vi "1D Weighted-Unweighted Chi2.vi"(8 "error in (no error)":errorcluster, 9 "Weight Array":dbl[](array[numeric]), 10 "Y Array":dbl[](array[numeric]), 11 "Fit Output":T1) -> (0 "error out":errorcluster, 3 "NL Fit Output":T1)   [LabVIEW 2021, in "Fits.lvlib"]
uses:
  Fits.lvlib
  Non-linear Fit Output v4.ctl
  Nonlinear Fit Method.ctl
  <vilib>/Analysis/Matrix/Datatypes/RealMatrix.ctl
  Convergence Criteria.ctl
  Non-linear Fitting Algorithm.ctl
  IRF(X)PSED/Fit Weights Type v2.ctl
  Graphs/XY Graph/XY Graph Plot Data.ctl
  <vilib>/Utility/error.llb/Error Cluster From Error Code.vi
  <vilib>/ErrorRing/Error Ring.xnode
  <vilib>/Analysis/Matrix/NI_Matrix.lvlib
  Graphs/XY Graph/XY Graph Add-Ons.lvlib
panel:
  # "see the AlliGator License on the block diagram (Ctrl+E or Window:Show Block Diagram)"
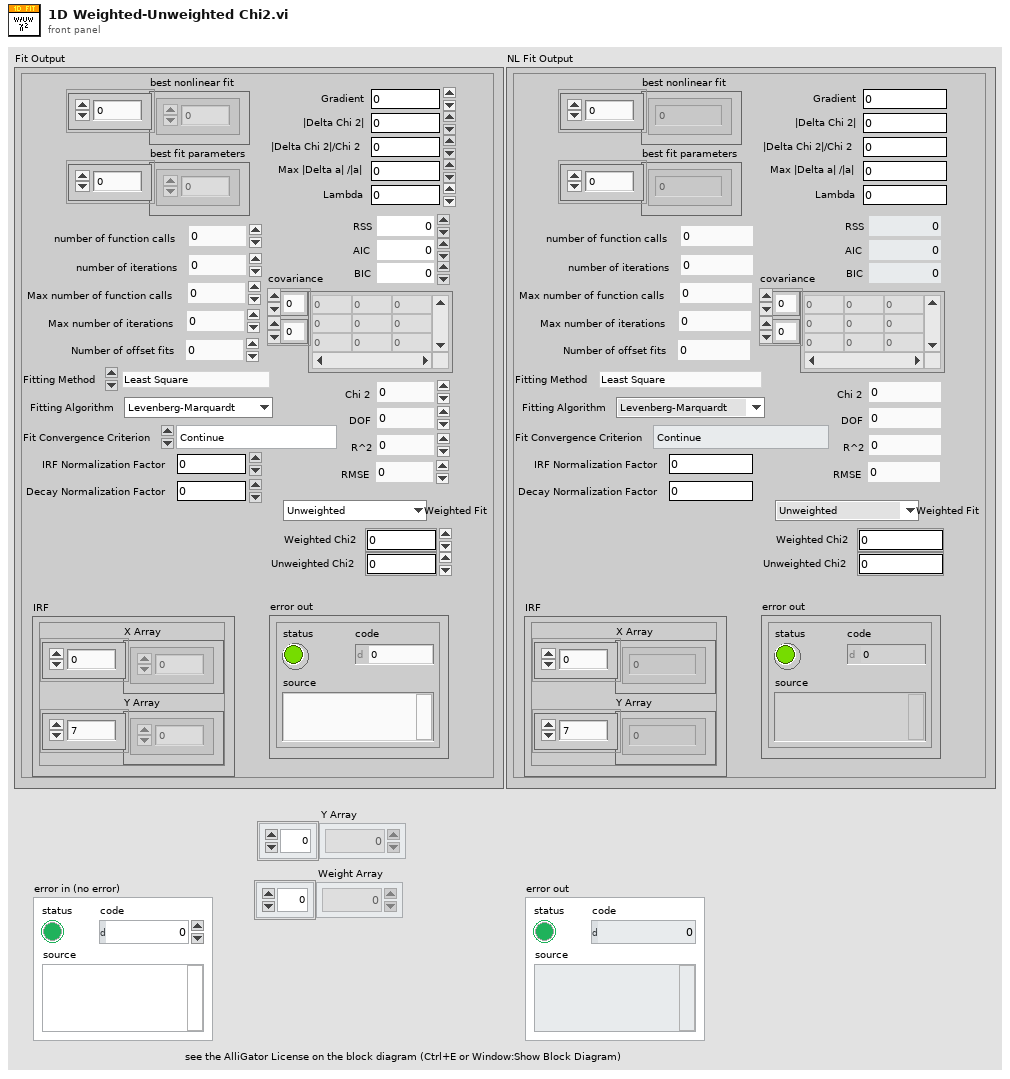
[diagram p1: front panel]
types:
  T1 = typedef "Fits.lvlib/Non-linear Fit Output v4.ctl" = cluster{"best nonlinear fit":dbl[], "best fit parameters":dbl[], "R^2":dbl, "RMSE":dbl, "error out":errorcluster, "Fitting Method":T2, "number of function calls":i32, "number of iterations":i32, "covariance":T3, "Chi 2":dbl, "DOF":i32, "Fit Convergence Criterion":T4, "Fitting Algorithm":T5, "Weighted Fit":T6, "Gradient":dbl, "|Delta Chi 2|":dbl, "|Delta Chi 2|/Chi 2":dbl, "Max |Delta a| /|a|":dbl, "Lambda":dbl, "RSS":dbl, "AIC":dbl, "BIC":dbl, "Max number of function calls":i32, "Max number of iterations":i32, "IRF":T7, "IRF Normalization Factor":dbl, "Decay Normalization Factor":dbl, "Number of offset fits":i32, "Weighted Chi2":dbl, "Unweighted Chi2":dbl}
  T2 = typedef "Fits.lvlib/Nonlinear Fit Method.ctl" = enum16{"Least Square", "Least Absolute Residual", "Bisquare", "MLE"}
  T3 = typedef "NI_Matrix.lvlib/RealMatrix.ctl" = dbl[][]
  T4 = typedef "Fits.lvlib/Convergence Criteria.ctl" = enum16{"Continue", "Tolerances Exceeded", "Max Time Exceeded", "Max Iterations Exceeded", "Max Function Evaluations Exceeded", "Scale Range Exceeded"}
  T5 = typedef "Fits.lvlib/Non-linear Fitting Algorithm.ctl" = enum16{"Levenberg-Marquardt", "Trust-Region Dogleg"}
  T6 = typedef "Fits.lvlib/Fit Weights Type v2.ctl" = enum16{"Unweighted", "1/Variance (Neyman)", "1/Variance (Pearson)", "Best of All"}
  T7 = typedef "XY Graph Add-Ons.lvlib/XY Graph Plot Data.ctl" = cluster{"X Array":dbl[], "Y Array":dbl[]}
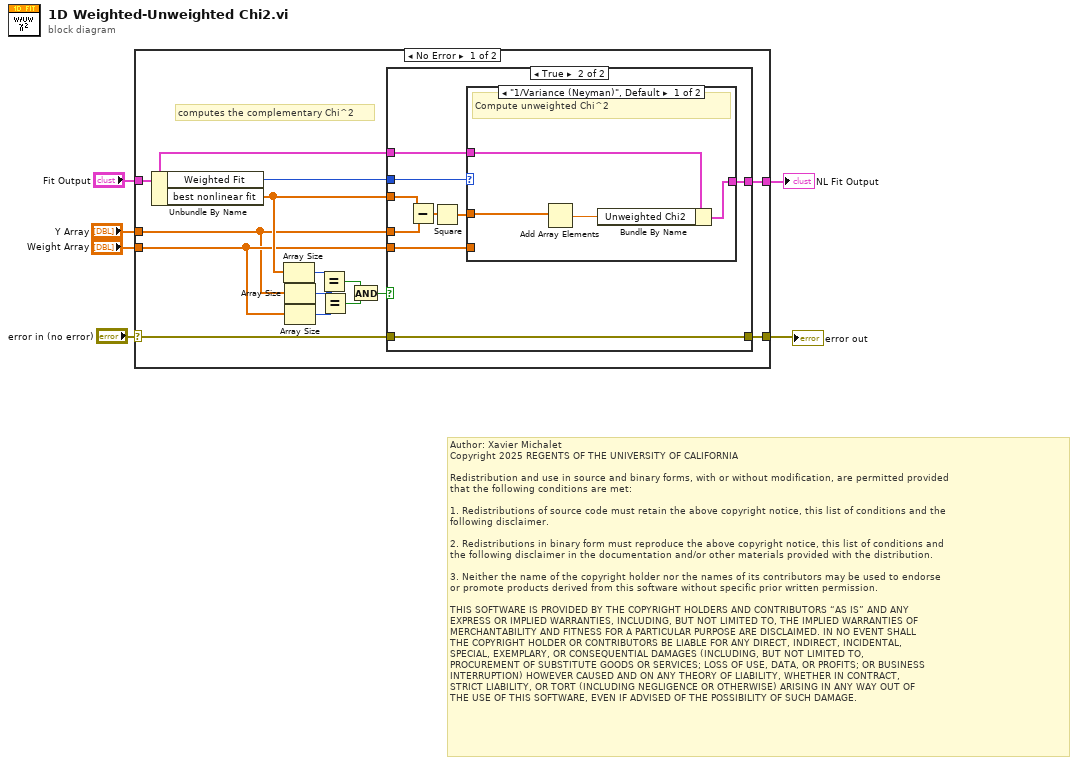
[diagram p0: block diagram]
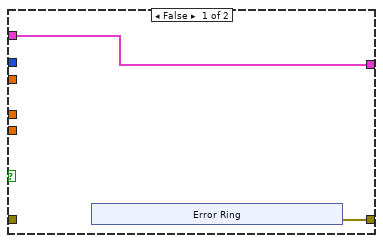
[diagram p2: hidden frame]
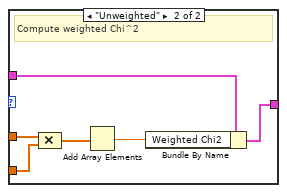
[diagram p3: hidden frame]
diagram:
  # "Author: Xavier Michalet\nCopyright 2025 REGENTS OF THE UNIVERSITY OF CALIFORNIA\n\nRedistribution and use in source and binary forms, with or without modification, are permitted provided\nthat the following conditions are met:\n\n1. Redistributions of source code must retain the above copyright notice, this list of conditions and the\nfollowing disclaimer.\n\n2. Redistributions in binary form must reproduce the above copyright notice, this list of conditions and\nthe following disclaimer in the documentation and/or other materials provided with the distribution.\n\n3. Neither the name of the copyright holder nor the names of its contributors may be used to endorse \nor promote products derived from this software without specific prior written permission.\n\nTHIS SOFTWARE IS PROVIDED BY THE COPYRIGHT HOLDERS AND CONTRIBUTORS “AS IS” AND ANY \nEXPRESS OR IMPLIED WARRANTIES, INCLUDING, BUT NOT LIMITED TO, THE IMPLIED WARRANTIES OF\nMERCHANTABILITY AND FITNESS FOR A PARTICULAR PURPOSE ARE DISCLAIMED. IN NO EVENT SHALL\nTHE COPYRIGHT HOLDER OR CONTRIBUTORS BE LIABLE FOR ANY DIRECT, INDIRECT, INCIDENTAL, \nSPECIAL, EXEMPLARY, OR CONSEQUENTIAL DAMAGES (INCLUDING, BUT NOT LIMITED TO, \nPROCUREMENT OF SUBSTITUTE GOODS OR SERVICES; LOSS OF USE, DATA, OR PROFITS; OR BUSINESS\nINTERRUPTION) HOWEVER CAUSED AND ON ANY THEORY OF LIABILITY, WHETHER IN CONTRACT, \nSTRICT LIABILITY, OR TORT (INCLUDING NEGLIGENCE OR OTHERWISE) ARISING IN ANY WAY OUT OF\nTHE USE OF THIS SOFTWARE, EVEN IF ADVISED OF THE POSSIBILITY OF SUCH DAMAGE."
  n1 = case shown="No Error" "error in (no error)" {
    selector: "error in (no error)" -> [w8 w47]
    tunnel: "Fit Output" -> [w19 w46]
    tunnel: [w18 w46] -> w5
    tunnel: "Weight Array" -> [w16 _]
    tunnel: "Y Array" -> [w14 _]
    tunnel: [w7 w47] -> w1
    frame No Error {
      # "computes the complementary Chi^2"
      n2 = Unbundle By Name(w19) -> ("Weighted Fit"=w20:T6, "best nonlinear fit"=w17:dbl[])
      n3 = Array Size(array=w17) -> (size(s)=w15:i32)
      n4 = Array Size(array=w14) -> (size(s)=w12:i32)
      n5 = Array Size(array=w16) -> (size(s)=w13:i32)
      n6 = Equal?(x=w15, y=w12) -> (x = y?=w11:bool)
      n7 = Equal?(x=w12, y=w13) -> (x = y?=w10:bool)
      n8 = And(x=w11, y=w10) -> (x .and. y?=w9:bool)
      n9 = case shown="True" w9 {
        tunnel: w20 -> [_ w35]
        tunnel: w19 -> [w22 w34]
        tunnel: [w22 w33] -> w18
        tunnel: w17 -> [_ w30]
        tunnel: w16 -> [_ w29]
        tunnel: w14 -> [_ w28]
        tunnel: w8 -> [_ w27]
        tunnel: [w21 w27] -> w7
        frame False {
          n10 = xnode "Error Ring"() -> ("error out"=w21:errorcluster)
        }
        frame True {
          n11 = Subtract(x=w30, y=w28) -> (x-y=w31:dbl[])
          n12 = Square(x=w31) -> (x^2=w32:dbl[])
          n13 = case shown="\"1/Variance (Neyman)\", Default" w35 {
            tunnel: w34 -> [w37 w43]
            tunnel: [w38 w44] -> w33
            tunnel: w29 -> [_ w40]
            tunnel: w32 -> [w36 w42]
            frame "1/Variance (Neyman)", Default {
              # "Compute unweighted Chi^2"
              n14 = Add Array Elements(numeric array=w36) -> (sum=w39:dbl)
              n15 = Bundle By Name(cluster=w37, "Unweighted Chi2"=w39) -> (w38:T1)
            }
            frame "Unweighted" {
              # "Compute weighted Chi^2"
              n16 = Compound Arithmetic op=MULTIPLY(w42, w40) -> (w41:dbl[])
              n17 = Add Array Elements(numeric array=w41) -> (sum=w45:dbl)
              n18 = Bundle By Name(cluster=w43, "Weighted Chi2"=w45) -> (w44:T1)
            }
          }
        }
      }
    }
    frame Error {
    }
  }
  "error out" <- w1
  "NL Fit Output" <- w5
